vi "PWM.vi"() -> ()   [LabVIEW 2011]
uses:
  <vilib>/robotics/Utilities/FPGA Utilities/Generate Digital Pulse (uSec).vi
  <vilib>/rvi/eio/common/nirviEmuTemplateMethod_errors.vi
  <vilib>/eio/EIONode/EIONode.xnode
  <vilib>/robotics/Utilities/FPGA Utilities/NI_Robotics_FPGA Utilities.lvlib
panel:
  in  "stop blink":bool
  in  "stop PWM":bool
  in  "pulse width (uSec)":u32=1500
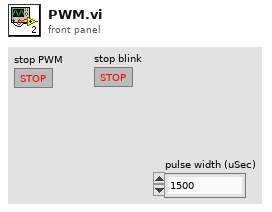
[diagram p1: front panel]
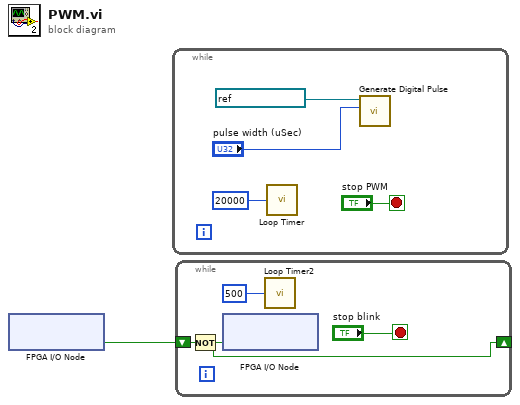
[diagram p0: block diagram]
diagram:
  n1 = xnode "FPGA I/O Node"() -> ("FPGA LED"=w1:bool)  [unwired: 1 in, 1 out]
  n2 = while {
    stop <- "stop PWM" stop-if-true
    n3 = call "Loop Timer"("Count(uSec)"=u32 20000) -> ()  [unwired: 1 out]
    n4 = call-poly <vilib>:"Generate Digital Pulse.vi"("pulse width (uSec)"="pulse width (uSec)", "FPGA digital output"=refnum<k21> "Mod4/DIO0") -> ()  [unwired: 10 in]
  }
  n5 = while {
    shift-right: [w6] -> _
    shift-left: w1 -> [w7]
    stop <- "stop blink" stop-if-true
    n6 = Not(x=w7) -> (.not. x?=w6:bool)
    n7 = xnode "FPGA I/O Node"("FPGA LED"=w6) -> ()  [unwired: 1 in, 1 out]
    n8 = call "Loop Timer2"("Count(mSec)"=u32 500 ("Count(uSec)")) -> ()  [unwired: 1 out]
  }
